vi "dummy reduced 2D.vi"(8 "error in (no error)":errorcluster) -> (0 "error out":errorcluster, 3 "Reduced 2D":dbl[][](array[numeric]))   [LabVIEW 2015]
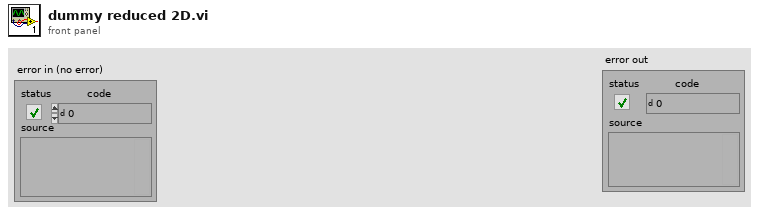
[diagram p1: front panel]
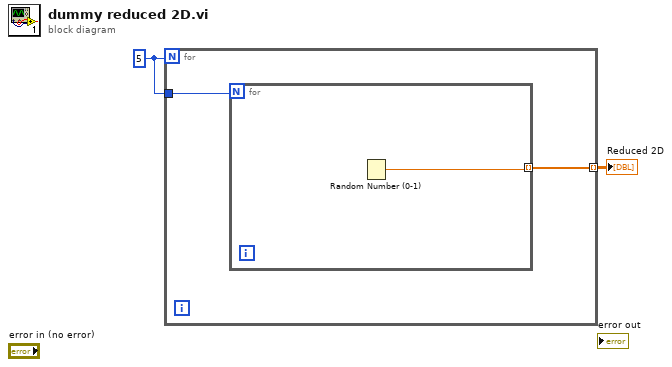
[diagram p0: block diagram]
diagram:
  w1 = 5
  n1 = for {
    N: w1 -> [_]
    tunnel: [w4] -> w2 mode=indexing
    tunnel: w1 -> [w3]
    n2 = for {
      N: w3 -> [_]
      tunnel: [w5] -> w4 mode=indexing
      n3 = Random Number (0-1)() -> (number: 0 to 1=w5:dbl)
    }
  }
  "Reduced 2D" <- w2
